vi "Two Processes One Stop.vi"() -> ()   [LabVIEW 2014]
doc: "This VI demonstrates two processes running in parallel."
panel:
  out "Input Data":dbl(graph)
  in  "stop":bool
  out "Value > 0?":bool
  out "Current Time":timestamp format="%<%I:%M:%S %p\n%x>T"
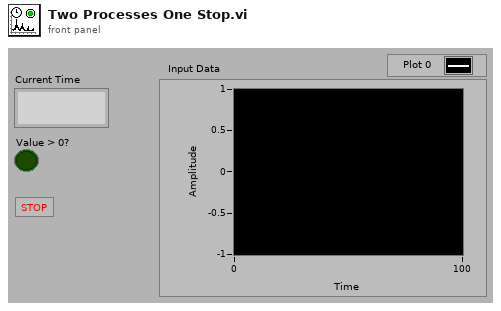
[diagram p1: front panel]
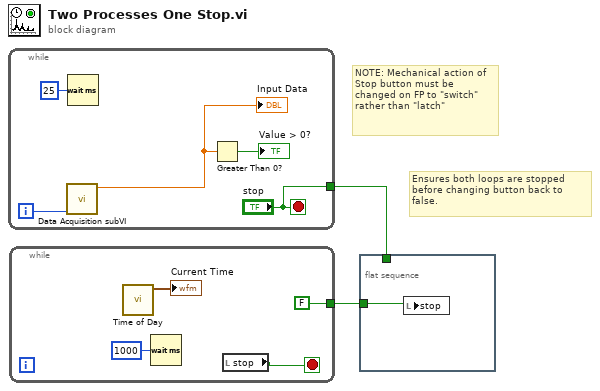
[diagram p0: block diagram]
diagram:
  # "Ensures both loops are stopped before changing button back to false."
  # "NOTE: Mechanical action of Stop button must be changed on FP to \"switch\" rather than \"latch\""
  n1 = while {
    tunnel: ["stop"] -> w1
    i -> [w5]
    stop <- "stop" stop-if-true
    n2 = call "Data Acquisition subVI.vi"("Numeric in"=w5) -> ("Numeric out"=w7:dbl)  [unwired: 10 in]
    "Input Data" <- w7
    n3 = Wait (ms)(milliseconds to wait=u32 25) -> ()  [unwired: 1 out]
    n4 = Greater Than 0?(x=w7) -> (x > 0?=→"Value > 0?":bool)
  }
  n5 = while {
    tunnel: [FALSE] -> w2
    stop <- w9 stop-if-true
    n6 = call "Time of Day.vi"() -> ("current time"=→"Current Time":timestamp)  [unwired: 11 in]
    n7 = Wait (ms)(milliseconds to wait=u32 1000) -> ()  [unwired: 1 out]
    n8 = local read "stop"() -> (w9:bool)
  }
  n9 = flat-sequence {
    tunnel: w2 -> [w12]
    tunnel: w1 -> [_]
    frame #0 {
      n10 = local write "stop"(w12) -> ()
    }
  }
